vi "FPGA Host.vi"() -> ()   [LabVIEW 2015]
uses:
  <vilib>/rvi/Emulation/niFpgaGetClockAttributes.vi
  <vilib>/rvi/Emulation/niFpgaSctlEmulationGetInTimedLoop.vi
  <vilib>/rvi/Emulation/niFpgaEmulationReportErrorSimple.vi
  Globals.vi
  <vilib>/rvi/Emulation/niFpgaProcessEmulError.vi
  <vilib>/rvi/Emulation/niFpgaCriticalErrorInLSC.vi
panel:
  out "Waveform DRAM done":bool=TRUE
  out "Errors":bool[](array[boolean])
  out "Total Waveform data points Indicator":u32
  out "Element address final":u32
  out "Waveform data points written final":u32
  in  "Total Waveform data points":u32
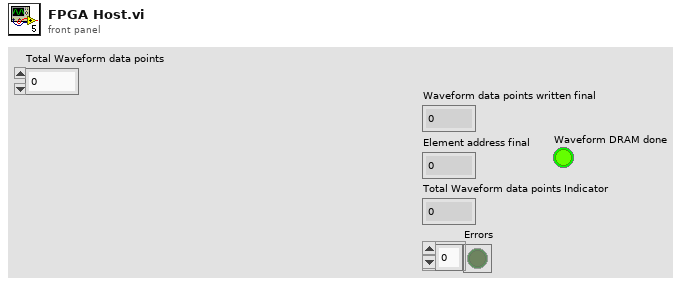
[diagram p1: front panel]
types:
  T1 = enum16{"Initialization", "Load Waveform", "Scanning", "Stop"}
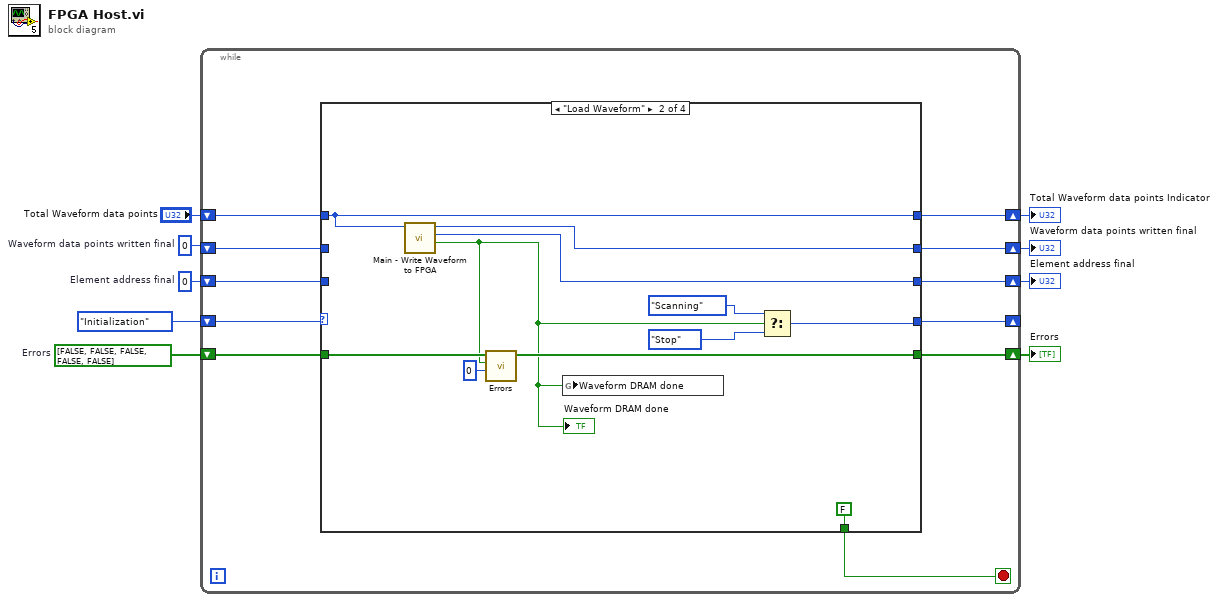
[diagram p0: block diagram]
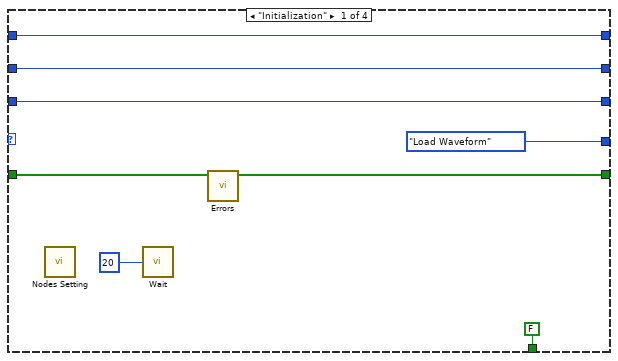
[diagram p2: hidden frame]
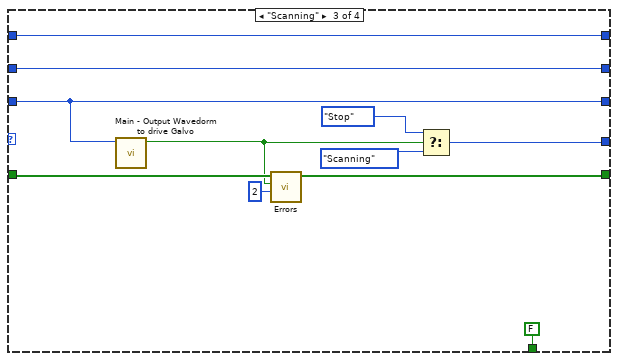
[diagram p3: hidden frame]
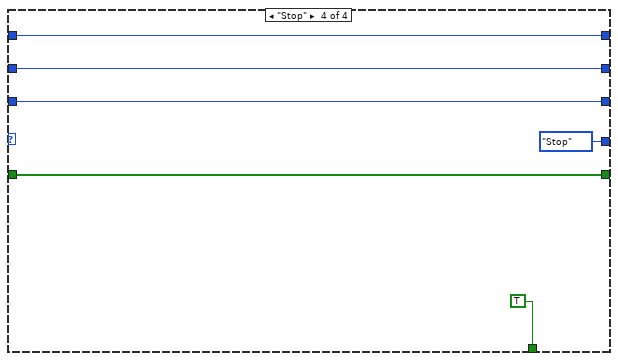
[diagram p4: hidden frame]
diagram:
  w3 = bool[] [FALSE, FALSE, FALSE, FALSE, FALSE]  # Errors
  w4 = u32 0  # Waveform data points written final
  w8 = u32 0  # Element address final
  n1 = while {
    shift-right: [w19] -> _
    shift-left: T1."Initialization" -> [w20]
    shift-right: [w18] -> w5
    shift-left: "Total Waveform data points" -> [w14]
    shift-right: [w16] -> w6
    shift-left: w8 -> [w15]
    shift-right: [w17] -> w7
    shift-left: w4 -> [w13]
    shift-right: [w12] -> w2
    shift-left: w3 -> [w11]
    stop <- w10 stop-if-true
    n2 = case shown="\"Load Waveform\"" w20 {
      tunnel: [T1."Load Waveform" w36 w41 T1."Stop" ("f")] -> w19
      tunnel: [w21 w34 w50 w56] -> w18
      tunnel: w14 -> [w21 w34 w50 w56]
      tunnel: [w22 w39 w48 w52] -> w17
      tunnel: [w26 w38 w49 w51] -> w16
      tunnel: w15 -> [w26 _ w49 w51]
      tunnel: w13 -> [w22 _ w48 w52]
      tunnel: [w25 w31 w46 w54] -> w12
      tunnel: w11 -> [w24 w33 w47 w54]
      tunnel: [FALSE FALSE FALSE TRUE] -> w10
      frame "Initialization" {
        n3 = call "Nodes Setting.vi"() -> ()  [unwired: 12 in]
        n4 = call "Wait"("Count(mSec)"=u32 20) -> ()  [unwired: 1 out]
        n5 = call "Errors.vi"("Errors in"=w24) -> ("Erros out"=w25:bool[])  [unwired: 10 in]
      }
      frame "Load Waveform" {
        n6 = call "Main - Write Waveform to FPGA.vi"("Total Waveform data points"=w34) -> ("All points written?"=w29:bool, "Element address final"=w38:u32, "Waveform data points written final"=w39:u32)  [unwired: 8 in]
        "Waveform DRAM done" <- w29
        n7 = call "Errors.vi"("Error ID"=0, "Done?"=w29, "Errors in"=w33) -> ("Erros out"=w31:bool[])  [unwired: 8 in]
        n8 = global write "Globals.vi" "Waveform DRAM done"(w29) -> ()
        n9 = Select(t=T1."Scanning", s=w29, f=T1."Stop") -> (s? t:f=w36:T1)
      }
      frame "Scanning" {
        n10 = call "Main - Output Wavedorm to drive Galvo.vi"("Element address final"=w49) -> ("Waveform Output Done"=w43:bool)  [unwired: 10 in]
        n11 = call "Errors.vi"("Error ID"=2, "Done?"=w43, "Errors in"=w47) -> ("Erros out"=w46:bool[])  [unwired: 8 in]
        n12 = Select(t=T1."Stop" ("f"), s=w43, f=T1."Scanning") -> (s? t:f=w41:T1)
      }
      frame "Stop" {
      }
    }
  }
  "Waveform data points written final" <- w7
  "Element address final" <- w6
  "Total Waveform data points Indicator" <- w5
  "Errors" <- w2
